vi "Open_Connection.vi"(7 "AccelNET.lvlib:TCP.lvclass":refnum<class "TCP.lvclass">, 8 "timeout ms (60000)":i32=60000, 9 "Write Port":i16, 10 "Read Port":i16, 11 "IP Address":string) -> (0 "Write Error":errorcluster, 1 "Read Error":errorcluster, 3 "AccelNET.lvlib:TCP.lvclass 2":refnum<class "TCP.lvclass">, 4 "Write ID":refnum<k5>, 5 "Read ID":refnum<k5>)   [LabVIEW 2012, in "AccelNET.lvlib" / "TCP.lvclass"]
uses:
  TCP.lvclass
  TCP.lvclass/TCP.ctl
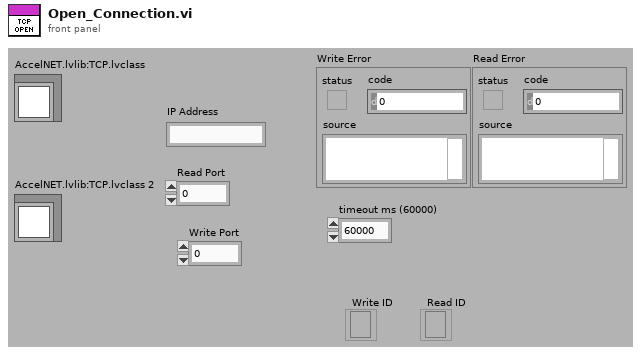
[diagram p1: front panel]
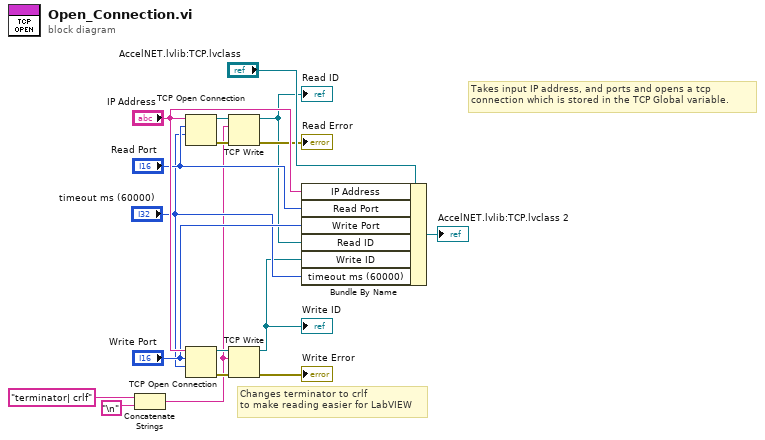
[diagram p0: block diagram]
diagram:
  # "Changes terminator to crlf\nto make reading easier for LabVIEW"
  # "Takes input IP address, and ports and opens a tcp\nconnection which is stored in the TCP Global variable."
  n1 = Concatenate Strings("terminator| crlf" ("data in"), "\n") -> (w1:string)
  n2 = TCP Open Connection(address="IP Address", remote port or service name="Read Port", timeout ms (60000)="timeout ms (60000)") -> (connection ID=w12:refnum<k5>, error out=w10:errorcluster)  [unwired: 2 in]
  n3 = TCP Open Connection(address="IP Address", remote port or service name="Write Port", timeout ms (60000)="timeout ms (60000)") -> (connection ID=w11:refnum<k5>, error out=w8:errorcluster)  [unwired: 2 in]
  n4 = TCP Write(connection ID=w12, data in=w1, error in (no error)=w10) -> (connection ID out=w5:refnum<k5>, error out=→"Read Error":errorcluster)  [unwired: 1 in, 1 out]
  "Read ID" <- w5
  n5 = TCP Write(connection ID=w11, data in=w1, error in (no error)=w8) -> (connection ID out=w4:refnum<k5>, error out=→"Write Error":errorcluster)  [unwired: 1 in, 1 out]
  "Write ID" <- w4
  n6 = Bundle By Name(cluster="AccelNET.lvlib:TCP.lvclass", "IP Address"="IP Address", "Read Port"="Read Port", "Write Port"="Write Port", "Read ID"=w5, "Write ID"=w4, "timeout ms (60000)"="timeout ms (60000)") -> (→"AccelNET.lvlib:TCP.lvclass 2":refnum<class "TCP.lvclass">)
